vi "remove_item_by_name.vi"(8 "error in (no error)":errorcluster, 10 "item_name":string, 11 "InlineTable in":refnum<class "InlineTable.lvclass">) -> (0 "error out":errorcluster, 2 "removed?":bool, 3 "InlineTable out":refnum<class "InlineTable.lvclass">)   [LabVIEW 2020, in "toml_edit.lvlib" / "InlineTable.lvclass"]
uses:
  InlineTable.lvclass
  InlineTable.lvclass/InlineTable.ctl
  dragon_toml_64.dll
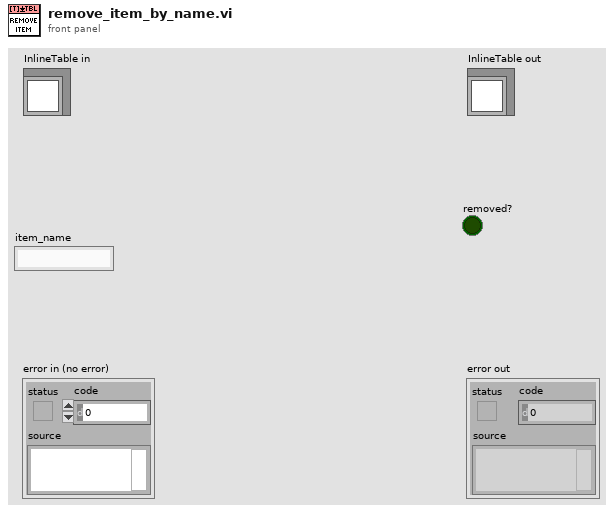
[diagram p1: front panel]
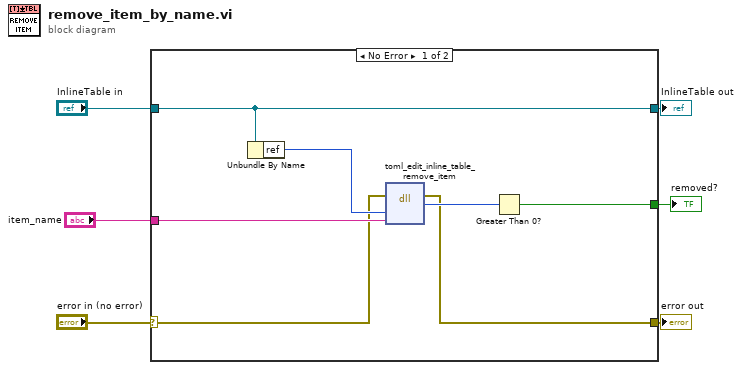
[diagram p0: block diagram]
diagram:
  n1 = case shown="No Error" "error in (no error)" {
    selector: "error in (no error)" -> [w8 w15]
    tunnel: [w7 w15] -> w5
    tunnel: [w10 w14] -> w3
    tunnel: "InlineTable in" -> [w10 w14]
    tunnel: [w11 _] -> w2
    tunnel: "item_name" -> [w9 _]
    frame No Error {
      n2 = Unbundle By Name(w10) -> ("ref"=w13:u64)
      n3 = dll-call lib="C:/Users/JamesMcNally/Documents/toml-edit-labview/lv_src/dragon_toml_*.*" fn="toml_edit_inline_table_remove_item"(error in=w8, "table_ref"=w13, "item_name"=w9) -> (error out=w7:errorcluster, "return"=w12:u64)  [unwired: 4 in, 1 out]
      n4 = Greater Than 0?(x=w12) -> (x > 0?=w11:bool)
    }
    frame Error {
    }
  }
  "error out" <- w5
  "InlineTable out" <- w3
  "removed?" <- w2
